vi "CheckState.vi"(8 "Error In":errorcluster, 10 "With sound?":bool, 11 "Astromech droid in":refnum<class "Astromech droid.lvclass">) -> (0 "Error Out":errorcluster, 3 "Astromech droid out":refnum<class "Astromech droid.lvclass">)   [LabVIEW 2021, in "Astromech droid.lvclass"]
uses:
  Astromech droid.lvclass
  Droid/Droid.lvclass
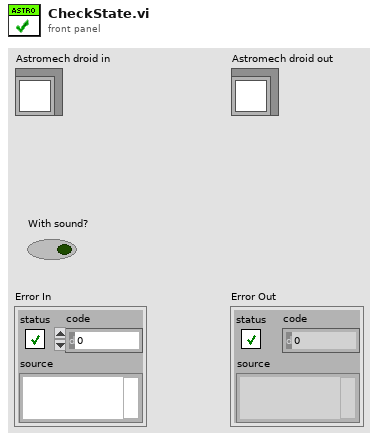
[diagram p1: front panel]
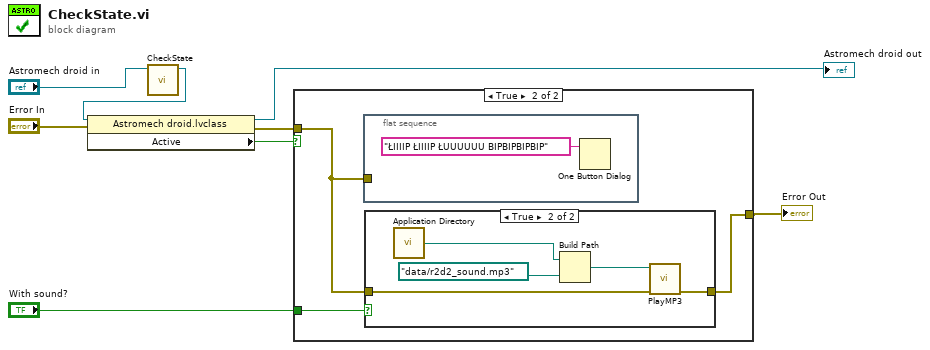
[diagram p0: block diagram]
diagram:
  n1 = call-parent "CheckState.vi"("Droid in"="Astromech droid in") -> ("Droid out"=w1:refnum<class "Astromech droid.lvclass">)  [unwired: 9 in, 1 out]
  n2 = property class="Astromech droid.lvclass"(reference=w1, error in="Error In") -> (reference out=→"Astromech droid out":refnum<class "Astromech droid.lvclass">, error out=w7:errorcluster, "Active"=w8:bool)
  n3 = case shown="True" w8 {
    tunnel: [w9 w12] -> w4
    tunnel: "With sound?" -> [_ w10]
    tunnel: w7 -> [w9 w11]
    frame False {
    }
    frame True {
      n4 = flat-sequence {
        tunnel: w11 -> [_]
        frame #0 {
          n5 = One Button Dialog(message="ŁIIIIP ŁIIIIP ŁUUUUUU BIPBIPBIPBIP") -> ()  [unwired: 1 in, 1 out]
        }
      }
      n6 = case shown="True" w10 {
        tunnel: w11 -> [w14 w16]
        tunnel: [w14 w15] -> w12
        frame False {
        }
        frame True {
          n7 = call <vilib>:"Application Directory.vi"() -> ("Application Directory"=w17:path)
          n8 = Build Path(base path=w17, name or relative path=path "data/r2d2_sound.mp3") -> (appended path=w19:path)
          n9 = call "PlayMP3.vi"("Error In"=w16, "Path"=w19) -> ("Error out"=w15:errorcluster)  [unwired: 9 in]
        }
      }
    }
  }
  "Error Out" <- w4
